vi "Automatic Teller Machine (ATM).vi"() -> ()   [LabVIEW 2025]
doc: "ATM main VI."
uses:
  Active User Data.ctl
  Queue Cluster.ctl
  States.ctl
  Account Balance Data Cluster.ctl
panel:
  in  "Enter":bool
  in  "User Input":string
  in  "Right Buttons":T1
  out "Right Menu":T2
  in  "Left Buttons":T1
  out "Left Menu":T2
  in  "Card Simulator":bool
  out "ATM Messages":string
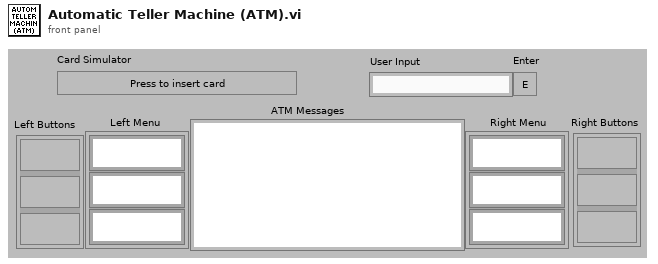
[diagram p1: front panel]
types:
  T1 = cluster{"Func Button":bool, "Func Button 2":bool, "Func Button 3":bool}
  T2 = cluster{"RFS String":string, "RFS String 2":string, "RFS String 3":string}
  T3 = typedef "Active User Data.ctl" = cluster{"Name":string, "Account Balance":dbl, "PIN":string}
  T4 = cluster{"RFS String":refnum<vi>, "RFS String 2":refnum<vi>, "RFS String 3":refnum<vi>}
  T5 = cluster{"Func Button":refnum<vi>, "Func Button 2":refnum<vi>, "Func Button 3":refnum<vi>}
  T6 = typedef "Queue Cluster.ctl" = cluster{"States":T7, "Data":variant}
  T7 = typedef "States.ctl" = enum16{"Withdraw", "Update Account Balance", "Deposit", "Balance Inquiry", "Verify Account", "Enable Account Actions", "Collect User Input", "Exit", "Init"}
  T8 = cluster{"Left Menu Strings":cluster{"RFS String":refnum<vi>, "RFS String 2":refnum<vi>, "RFS String 3":refnum<vi>}, "Right Menu Strings":cluster{"RFS String":refnum<vi>, "RFS String 2":refnum<vi>, "RFS String 3":refnum<vi>}, "Card Simulator":refnum<vi>, "Enter":refnum<vi>, "User Input":refnum<vi>, "Left Menu Button Refs":cluster{"Func Button":refnum<vi>, "Func Button 2":refnum<vi>, "Func Button 3":refnum<vi>}, "Right Menu Button Refs":cluster{"Func Button":refnum<vi>, "Func Button 2":refnum<vi>, "Func Button 3":refnum<vi>}}
  T9 = enum8{"Enabled", "Disabled", "Disabled and Grayed Out"}
  T10 = cluster{"User Input":string, "f":enum16{"Add", "Subtract"}}
  T11 = typedef "Account Balance Data Cluster.ctl" = cluster{"User Input":string, "Process":enum16{"Add", "Subtract"}}
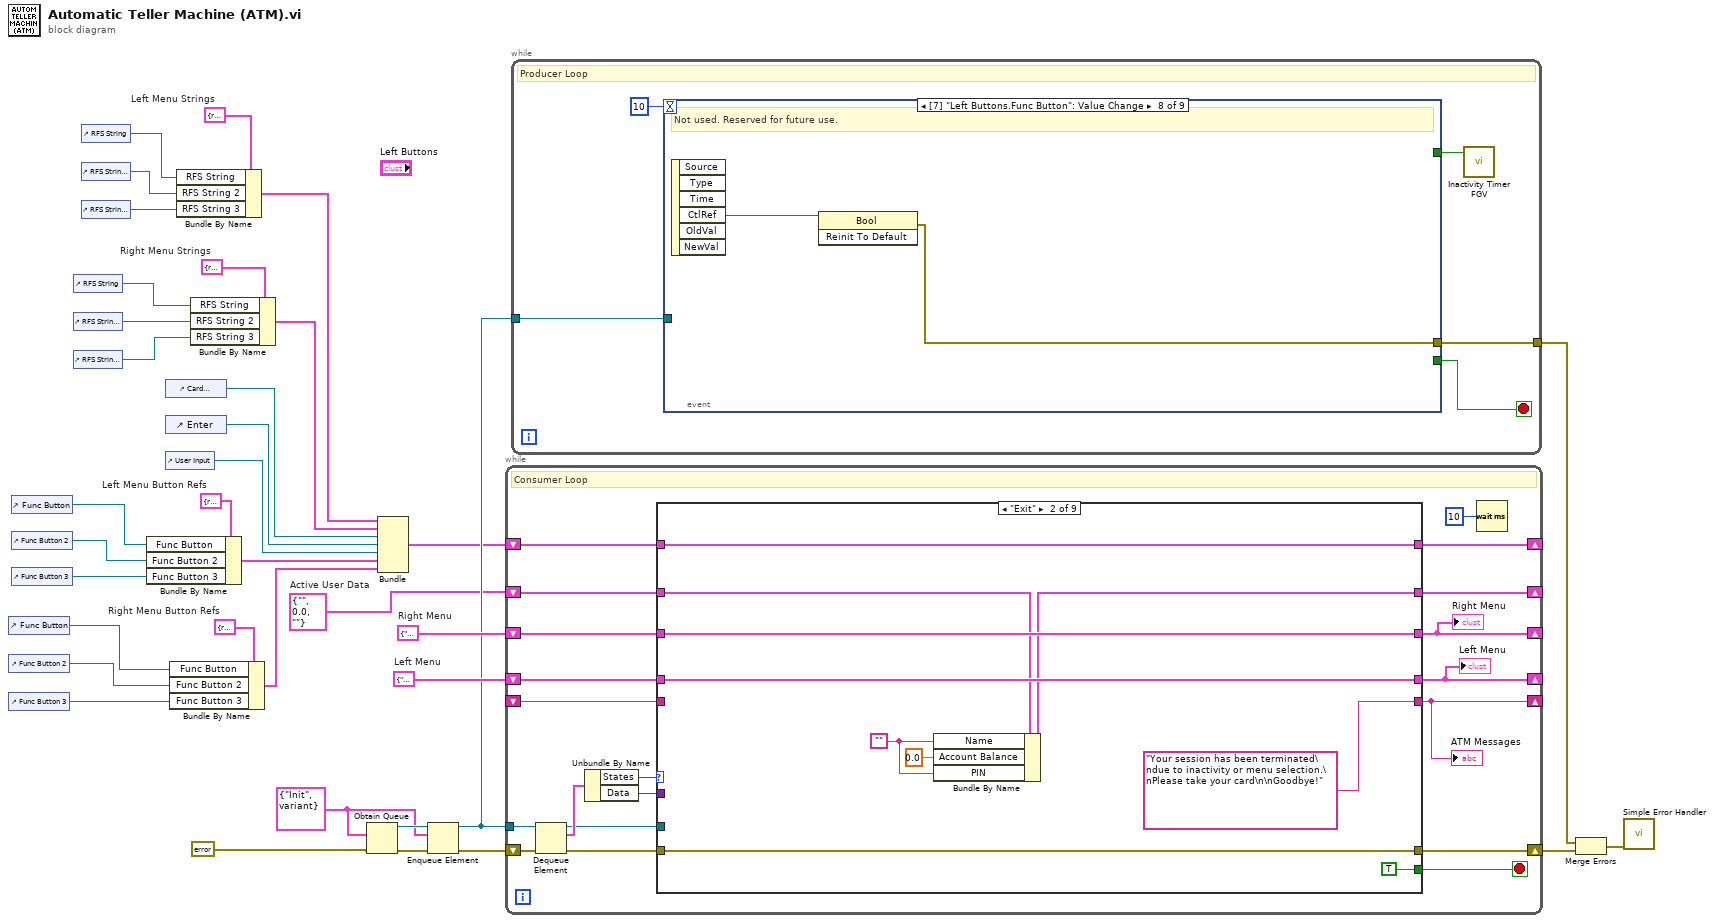
[diagram p0: block diagram]
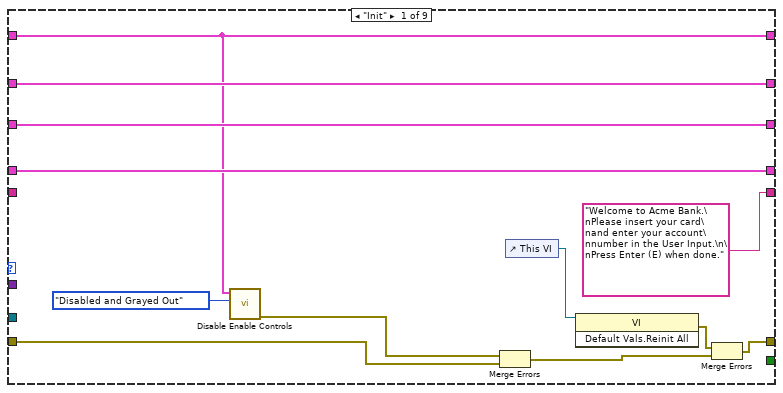
[diagram p2: hidden frame]
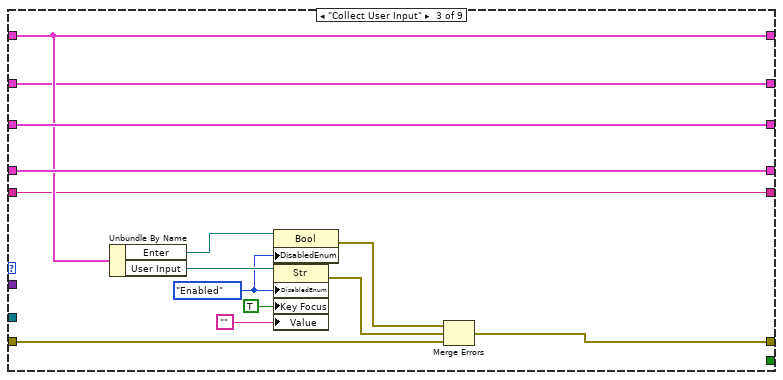
[diagram p3: hidden frame]
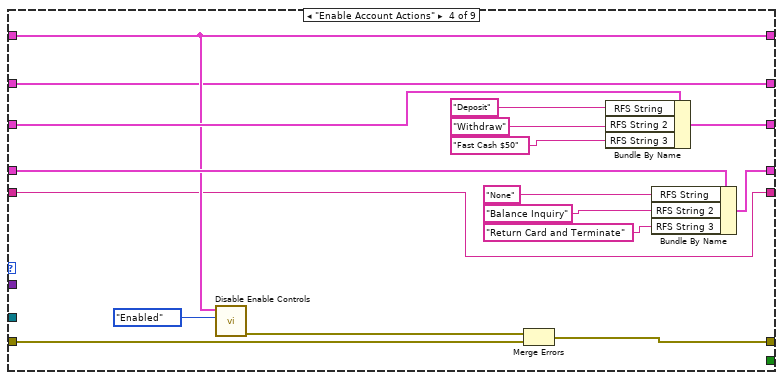
[diagram p4: hidden frame]
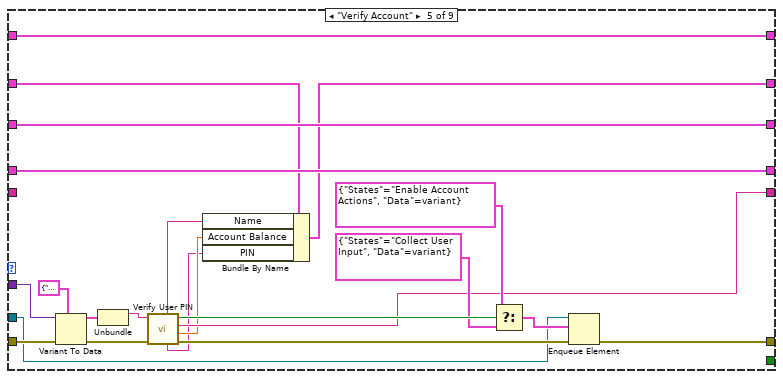
[diagram p5: hidden frame]
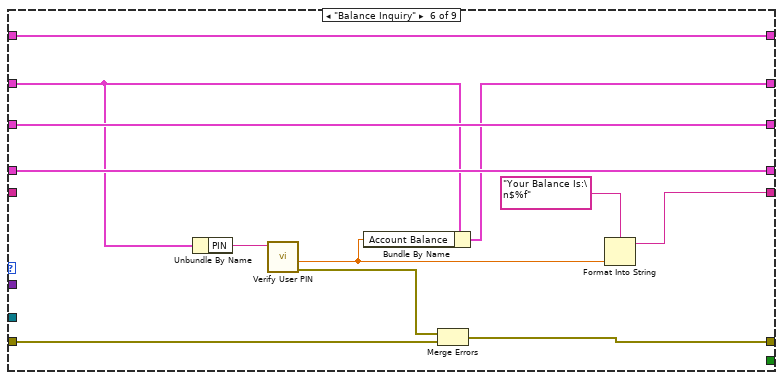
[diagram p6: hidden frame]
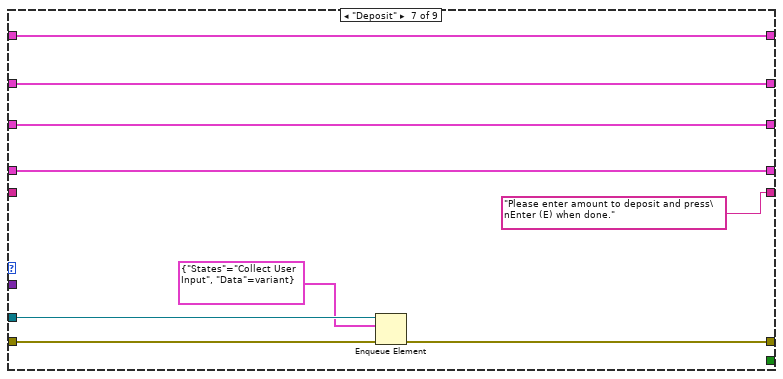
[diagram p7: hidden frame]
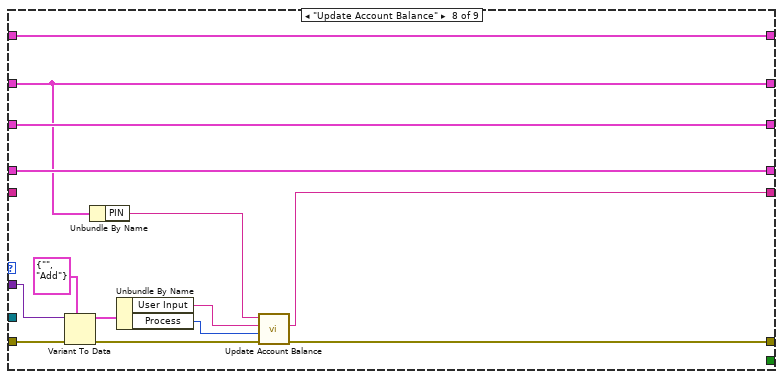
[diagram p8: hidden frame]
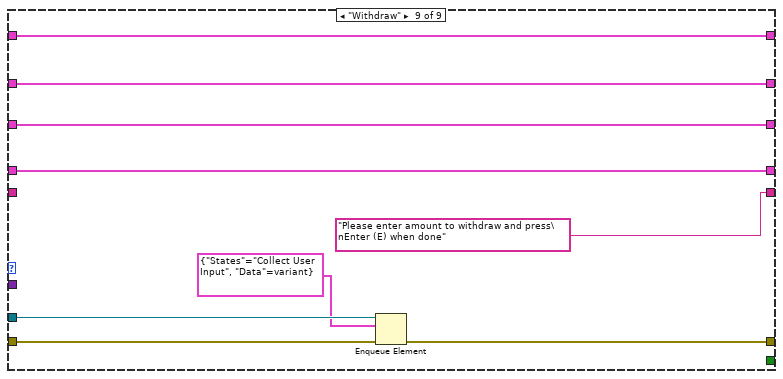
[diagram p9: hidden frame]
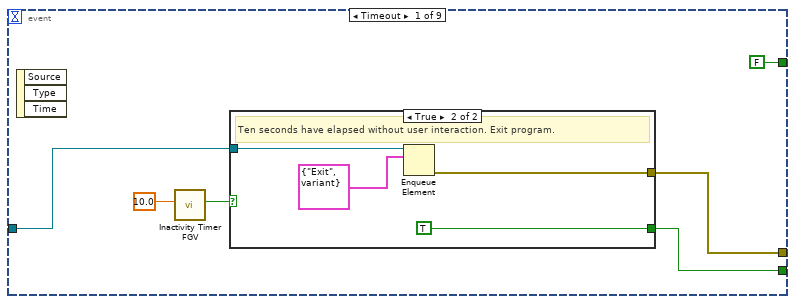
[diagram p10: hidden frame]
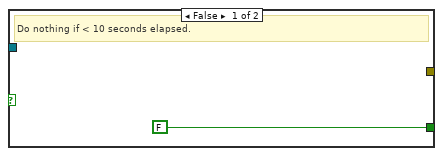
[diagram p11: hidden frame]
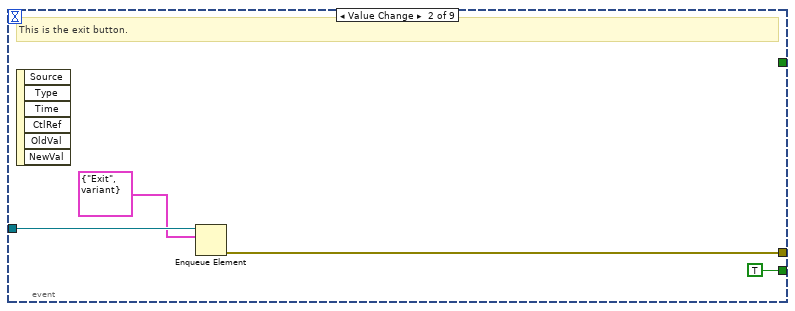
[diagram p12: hidden frame]
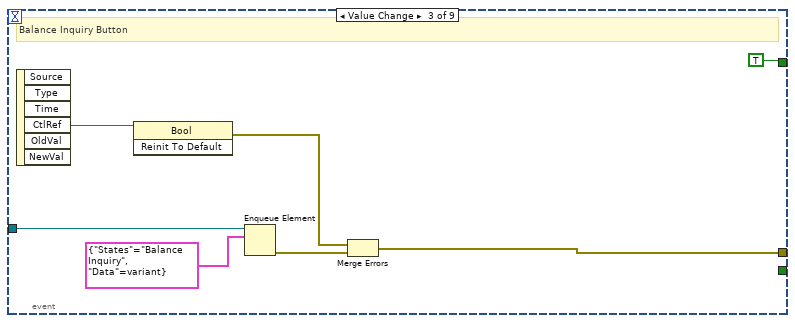
[diagram p13: hidden frame]
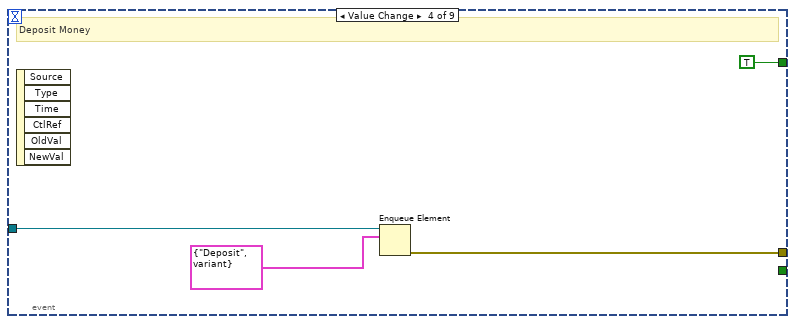
[diagram p14: hidden frame]
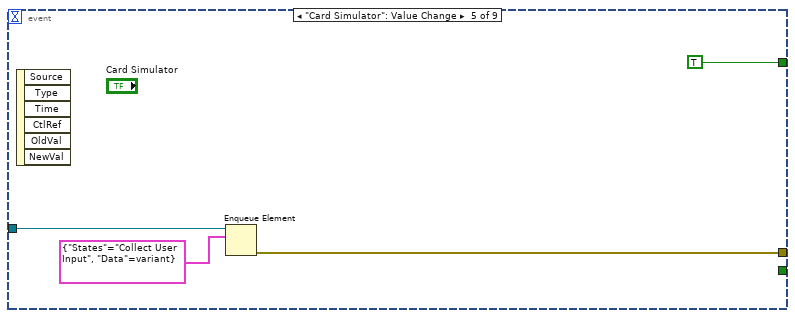
[diagram p15: hidden frame]
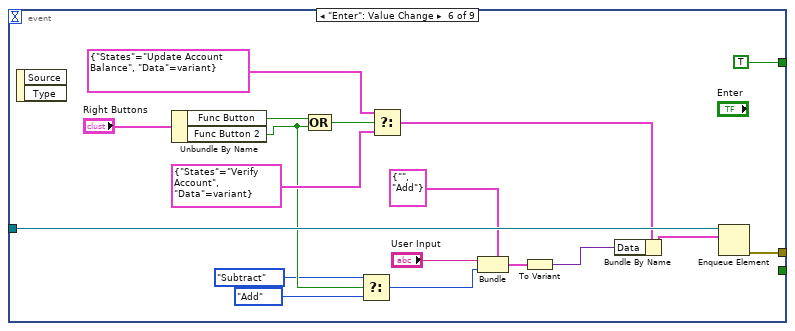
[diagram p16: hidden frame]
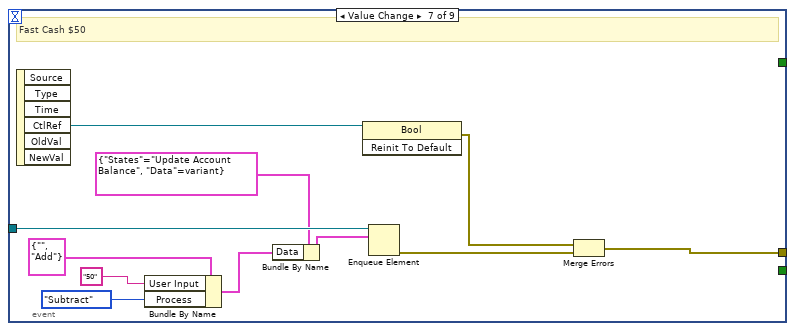
[diagram p17: hidden frame]
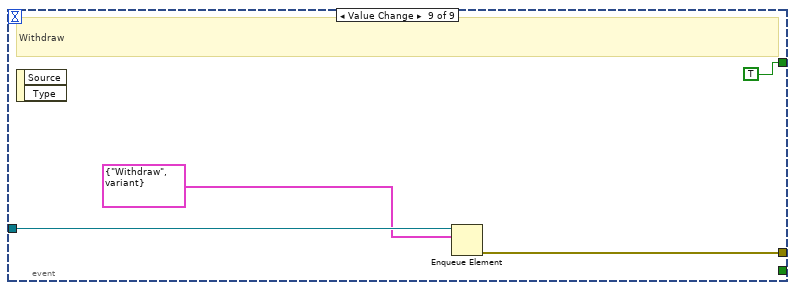
[diagram p18: hidden frame]
diagram:
  w2 = T3 {"Name"="", "Account Balance"=0.0, "PIN"=""}  # Active User Data
  w6 = T2 {"RFS String"="", "RFS String 2"="", "RFS String 3"=""}  # Left Menu
  w8 = T4 {"RFS String"=refnum, "RFS String 2"=refnum, "RFS String 3"=refnum}  # Right Menu Strings
  w13 = T4 {"RFS String"=refnum, "RFS String 2"=refnum, "RFS String 3"=refnum}  # Left Menu Strings
  w17 = T2 {"RFS String"="", "RFS String 2"="", "RFS String 3"=""}  # Right Menu
  w24 = T5 {"Func Button"=refnum, "Func Button 2"=refnum, "Func Button 3"=refnum}  # Right Menu Button Refs
  w28 = T5 {"Func Button"=refnum, "Func Button 2"=refnum, "Func Button 3"=refnum}  # Left Menu Button Refs
  w33 = T6 {"States"=enum."Init", "Data"=variant}
  n1 = control-ref of="Func Button"() -> (w27:refnum<vi>)
  n2 = control-ref of="Func Button 2"() -> (w26:refnum<vi>)
  n3 = control-ref of="Func Button 3"() -> (w25:refnum<vi>)
  n4 = control-ref of="Func Button"() -> (w30:refnum<vi>)
  n5 = control-ref of="Func Button 2"() -> (w31:refnum<vi>)
  n6 = control-ref of="Func Button 3"() -> (w29:refnum<vi>)
  n7 = control-ref of="RFS String"() -> (w11:refnum<vi>)
  n8 = control-ref of="RFS String 2"() -> (w10:refnum<vi>)
  n9 = control-ref of="RFS String 3"() -> (w9:refnum<vi>)
  n10 = control-ref of="RFS String"() -> (w16:refnum<vi>)
  n11 = control-ref of="RFS String 2"() -> (w15:refnum<vi>)
  n12 = control-ref of="RFS String 3"() -> (w14:refnum<vi>)
  n13 = Bundle By Name(cluster=w28, "Func Button"=w30, "Func Button 2"=w31, "Func Button 3"=w29) -> (w20:T5)
  n14 = control-ref of="Card Simulator"() -> (w23:refnum<vi>)
  n15 = control-ref of="Enter"() -> (w22:refnum<vi>)
  n16 = control-ref of="User Input"() -> (w21:refnum<vi>)
  n17 = Bundle By Name(cluster=w24, "Func Button"=w27, "Func Button 2"=w26, "Func Button 3"=w25) -> (w19:T5)
  n18 = Bundle By Name(cluster=w13, "RFS String"=w16, "RFS String 2"=w15, "RFS String 3"=w14) -> (w12:T4)
  n19 = Bundle By Name(cluster=w8, "RFS String"=w11, "RFS String 2"=w10, "RFS String 3"=w9) -> (w7:T4)
  n20 = Obtain Queue(element data type=w33, error in (no error)=errorcluster {"status"=FALSE, "code"=0, "source"=""}) -> (queue out=w36:refnum<queue>, error out=w35:errorcluster)  [unwired: 3 in, 1 out]
  n21 = Bundle("Left Menu Strings"=w12, "Right Menu Strings"=w7, "Card Simulator"=w23, "Enter"=w22, "User Input"=w21, "Left Menu Button Refs"=w20, "Right Menu Button Refs"=w19) -> (w1:T8)  [unwired: 1 in]
  n22 = Enqueue Element(queue=w36, element=w33, error in (no error)=w35) -> (queue out=w5:refnum<queue>, error out=w4:errorcluster)  [unwired: 1 in, 1 out]
  n23 = while {
    tunnel: w5 -> [w53]
    shift-right: [w48] -> _
    shift-left: w1 -> [w39]
    shift-right: [w46] -> _
    shift-left: w6 -> [w47]
    shift-right: [w44] -> _
    shift-left: w17 -> [w45]
    shift-right: [w42] -> _
    shift-left: _ -> [w41]
    shift-right: [w55] -> w34
    shift-left: w4 -> [w56]
    shift-right: [w37] -> _
    shift-left: w2 -> [w38]
    stop <- w49 stop-if-true
    # "Consumer Loop"
    n24 = Dequeue Element(queue=w53, error in (no error)=w56) -> (queue out=w43:refnum<queue>, element=w52:T6, error out=w54:errorcluster)  [unwired: 1 in, 1 out]
    n25 = Unbundle By Name(w52) -> ("States"=w51:T7, "Data"=w50:variant)
    n26 = case shown="\"Exit\"" w51 {
      tunnel: w54 -> [w68 w73 w92 w109 w128 w143 w152 w166 w175]
      tunnel: [w66 w73 w81 w97 w119 w135 w146 w158 w169] -> w55
      tunnel: w50 -> [_ _ _ _ w126 _ _ w162 _]
      tunnel: [_ TRUE _ _ _ _ _ _ _] -> w49
      tunnel: ["Welcome to Acme Bank.\nPlease insert your card\nand enter your account\nnumber in the User Input.\n\nPress Enter (E) when done." "Your session has been terminated\ndue to inactivity or menu selection.\nPlease take your card\n\nGoodbye!" w83 w95 w118 w139 "Please enter amount to deposit and press\nEnter (E) when done." ("ATM Message") w154 "Please enter amount to withdraw and press\nEnter (E) when done" ("ATM Message")] -> w42
      tunnel: w39 -> [w59 w76 w89 w98 w131 w138 w147 w165 w174]
      tunnel: [w59 w76 w89 w98 w131 w138 w147 w165 w174] -> w48
      tunnel: w47 -> [w65 w75 w91 w108 w130 w142 w151 w164 w173]
      tunnel: [w65 w75 w91 w104 w130 w142 w151 w164 w173] -> w46
      tunnel: w45 -> [w64 w74 w90 w103 w129 w141 w150 w163 w172]
      tunnel: [w64 w74 w90 w99 w129 w141 w150 w163 w172] -> w44
      tunnel: w43 -> [_ _ _ _ w120 _ w145 _ w168]
      tunnel: w41 -> [_ _ w83 w95 _ _ _ _ _]
      tunnel: w38 -> [w60 w72 w82 w94 w117 w137 w149 w161 w171]
      tunnel: [w60 w71 w82 w94 w116 w133 w149 w161 w171] -> w37
      frame "Init" {
        n27 = call "Disable Enable Controls.vi"("Disable or Enable"=T9."Disabled and Grayed Out", "Cluster"=w59) -> ("error out"=w57:errorcluster)  [unwired: 9 in]
        n28 = Merge Errors(w57, w68) -> (w61:errorcluster)
        n29 = control-ref of="This VI"() -> (w63:refnum<vi>)
        n30 = invoke on="Invoke Node" class="VI" method="Default Vals.Reinit All"(reference=w63) -> (error out=w62:errorcluster)  [unwired: 2 in, 2 out]
        n31 = Merge Errors(w62, w61) -> (w66:errorcluster)
      }
      frame "Exit" {
        w70 = "" ("Name")
        n32 = Bundle By Name(cluster=w72, "Name"=w70, "Account Balance"=0.0, "PIN"=w70) -> (w71:T3)
      }
      frame "Collect User Input" {
        w85 = T9."Enabled" ("Disabled")
        n33 = Unbundle By Name(w89) -> ("Enter"=w86:refnum<vi>, "User Input"=w88:refnum<vi>)
        n34 = property on="Property Node" class="Bool"(reference=w86, "DisabledEnum"=w85) -> (error out=w79:errorcluster)  [unwired: 1 in, 1 out]
        n35 = property on="Property Node" class="Str"(reference=w88, "DisabledEnum"=w85, "Key Focus"=TRUE ("Selected"), "Value"="" ("Empty String Constant")) -> (error out=w80:errorcluster)  [unwired: 1 in, 1 out]
        n36 = Merge Errors(w79, w80, w92) -> (w81:errorcluster)
      }
      frame "Enable Account Actions" {
        n37 = call "Disable Enable Controls.vi"("Disable or Enable"=T9."Enabled", "Cluster"=w98) -> ("error out"=w96:errorcluster)  [unwired: 9 in]
        n38 = Merge Errors(w96, w109) -> (w97:errorcluster)
        n39 = Bundle By Name(cluster=w103, "RFS String"="Deposit" ("Right Menu.RFS String"), "RFS String 2"="Withdraw" ("Right Menu.RFS String 2"), "RFS String 3"="Fast Cash $50" ("Right Menu.RFS String 3")) -> (w99:T2)
        n40 = Bundle By Name(cluster=w108, "RFS String"="None" ("Left Menu.RFS String"), "RFS String 2"="Balance Inquiry" ("Left Menu.RFS String 2"), "RFS String 3"="Return Card and Terminate" ("Left Menu.RFS String 3")) -> (w104:T2)
      }
      frame "Verify Account" {
        n41 = Variant To Data(error in=w128, type=T10 {"User Input"="", "f"=enum."Add"} ("cluster"), Variant=w126) -> (data=w111:T10, error out=w127:errorcluster)
        n42 = Unbundle(w111) -> ("User Input"=w110:string)  [unwired: 1 out]
        n43 = call "Verify User PIN.vi"("error in (no error)"=w127, "PIN"=w110) -> ("error out"=w121:errorcluster, "Account Balance"=w114:dbl, "ATM Message"=w118:string, "Verified?"=w124:bool, "User PIN"=w113:string, "Account Holder"=w115:string)  [unwired: 4 in]
        n44 = Bundle By Name(cluster=w117, "Name"=w115, "Account Balance"=w114, "PIN"=w113) -> (w116:T3)
        n45 = Select(t=T6 {"States"=enum."Enable Account Actions", "Data"=variant}, s=w124, f=T6 {"States"=enum."Collect User Input", "Data"=variant}) -> (s? t:f=w122:T6)
        n46 = Enqueue Element(queue=w120, element=w122, error in (no error)=w121) -> (error out=w119:errorcluster)  [unwired: 1 in, 2 out]
      }
      frame "Balance Inquiry" {
        n47 = Unbundle By Name(w137) -> ("PIN"=w136:string)
        n48 = call "Verify User PIN.vi"("PIN"=w136) -> ("error out"=w134:errorcluster, "Account Balance"=w132:dbl)  [unwired: 5 in, 4 out]
        n49 = Bundle By Name(cluster=w137, "Account Balance"=w132) -> (w133:T3)
        n50 = Merge Errors(w134, w143) -> (w135:errorcluster)
        n51 = Format Into String(format string="Your Balance Is:\n$%f", w132) -> (resulting string=w139:string)  [unwired: 2 in, 1 out]
      }
      frame "Deposit" {
        n52 = Enqueue Element(queue=w145, element=T6 {"States"=enum."Collect User Input", "Data"=variant}, error in (no error)=w152) -> (error out=w146:errorcluster)  [unwired: 1 in, 2 out]
      }
      frame "Update Account Balance" {
        n53 = Variant To Data(error in=w166, type=T11 {"User Input"="", "Process"=enum."Add"} ("Update Account Balance Data Cluster"), Variant=w162) -> (data=w157:T11, error out=w159:errorcluster)
        n54 = Unbundle By Name(w161) -> ("PIN"=w160:string)
        n55 = Unbundle By Name(w157) -> ("User Input"=w155:string, "Process"=w156:enum16{"Add", "Subtract"})
        n56 = call "Update Account Balance.vi"("error in (no error)"=w159, "Add or Subtract"=w156, "Amount"=w155, "PIN"=w160) -> ("error out"=w158:errorcluster, "Message"=w154:string)  [unwired: 6 in]
      }
      frame "Withdraw" {
        n57 = Enqueue Element(queue=w168, element=T6 {"States"=enum."Collect User Input", "Data"=variant}, error in (no error)=w175) -> (error out=w169:errorcluster)  [unwired: 1 in, 2 out]
      }
    }
    "ATM Messages" <- w42
    "Left Menu" <- w46
    "Right Menu" <- w44
    n58 = Wait (ms)(milliseconds to wait=u32 10) -> ()  [unwired: 1 out]
  }
  n59 = while {
    tunnel: w5 -> [w179]
    tunnel: [w180] -> w32
    stop <- w177 stop-if-true
    # "Producer Loop"
    n60 = event shown="[7] \"Left Buttons.Func Button\": Value Change" {
      selector: _ -> [_ _ _ _ _ _ _ _ _]
      dyn-events: _ -> [_ _ _ _ _ _ _ _ _]
      timeout: 10 -> [_ _ _ _ _ _ _ _ _]
      tunnel: w179 -> [w184 w195 w202 w206 w210 w228 w239 _ w245]
      tunnel: [w183 w193 w197 w205 w209 w227 w230 w240 w244] -> w180
      tunnel: [w182 TRUE _ _ _ _ _ _ _] -> w177
      tunnel: [FALSE ("Reset") _ TRUE ("Reset") TRUE ("Reset") TRUE ("Reset") TRUE ("Reset") _ _ TRUE ("Reset")] -> w176
      event Timeout {
        n61 = event-data() -> ()  [unwired: 1 in, 3 out]
        n62 = call "Inactivity Timer FGV.vi"("Time Target (s)"=10.0) -> ("Time has Elapsed"=w186:bool)  [unwired: 9 in, 1 out]
        n63 = case shown="True" w186 {
          tunnel: [FALSE TRUE] -> w182
          tunnel: w184 -> [_ w191]
          tunnel: [_ w189] -> w183
          frame False {
            # "Do nothing if < 10 seconds elapsed."
          }
          frame True {
            # "Ten seconds have elapsed without user interaction. Exit program."
            n64 = Enqueue Element(queue=w191, element=T6 {"States"=enum."Exit", "Data"=variant}) -> (error out=w189:errorcluster)  [unwired: 2 in, 2 out]
          }
        }
      }
      event "Left Buttons.Func Button 3": Value Change {
        # "This is the exit button."
        n65 = event-data() -> ()  [unwired: 1 in, 6 out]
        n66 = Enqueue Element(queue=w195, element=T6 {"States"=enum."Exit", "Data"=variant} ("Queue Cluster")) -> (error out=w193:errorcluster)  [unwired: 2 in, 2 out]
      }
      event "Left Buttons.Func Button 2": Value Change {
        # "Balance Inquiry Button"
        n67 = event-data() -> ("CtlRef"=w198:refnum<vi>)  [unwired: 1 in, 5 out]
        n68 = invoke on="Invoke Node" class="Bool" method="Reinit To Default"(reference=w198) -> (error out=w196:errorcluster)  [unwired: 2 in, 2 out]
        n69 = Enqueue Element(queue=w202, element=T6 {"States"=enum."Balance Inquiry", "Data"=variant}) -> (error out=w201:errorcluster)  [unwired: 2 in, 2 out]
        n70 = Merge Errors(w196, w201) -> (w197:errorcluster)
      }
      event "Right Buttons.Func Button": Value Change {
        # "Deposit Money"
        n71 = event-data() -> ()  [unwired: 1 in, 6 out]
        n72 = Enqueue Element(queue=w206, element=T6 {"States"=enum."Deposit", "Data"=variant}) -> (error out=w205:errorcluster)  [unwired: 2 in, 2 out]
      }
      event "Card Simulator": Value Change {
        n73 = event-data() -> ()  [unwired: 1 in, 6 out]
        n74 = Enqueue Element(queue=w210, element=T6 {"States"=enum."Collect User Input", "Data"=variant}) -> (error out=w209:errorcluster)  [unwired: 2 in, 2 out]
      }
      event "Enter": Value Change {
        n75 = event-data() -> ()  [unwired: 1 in, 2 out]
        n76 = Unbundle By Name("Right Buttons") -> ("Func Button"=w222:bool, "Func Button 2"=w216:bool)
        n77 = Compound Arithmetic op=OR(w222, w216) -> (w221:bool)
        n78 = Select(t=enum16{"Add", "Subtract"}."Subtract" ("Add or Subtract"), s=w216, f=enum16{"Add", "Subtract"}."Add") -> (s? t:f=w213:enum16{"Add", "Subtract"})
        n79 = Select(t=T6 {"States"=enum."Update Account Balance", "Data"=variant}, s=w221, f=T6 {"States"=enum."Verify Account", "Data"=variant}) -> (s? t:f=w218:T6)
        n80 = Bundle(cluster=T11 {"User Input"="", "Process"=enum."Add"} ("Update Account Balance Data Cluster"), "User Input"="User Input", "Process"=w213) -> (w217:T11)
        n81 = To Variant(anything=w217) -> (Variant=w225:variant)
        n82 = Bundle By Name(cluster=w218, "Data"=w225) -> (w226:T6)
        n83 = Enqueue Element(queue=w228, element=w226) -> (error out=w227:errorcluster)  [unwired: 2 in, 2 out]
      }
      event "Right Buttons.Func Button 3": Value Change {
        # "Fast Cash $50"
        n84 = event-data() -> ("CtlRef"=w231:refnum<vi>)  [unwired: 1 in, 5 out]
        n85 = Bundle By Name(cluster=T11 {"User Input"="", "Process"=enum."Add"}, "User Input"="50", "Process"=enum16{"Add", "Subtract"}."Subtract" ("f")) -> (w232:T11)
        n86 = Bundle By Name(cluster=T6 {"States"=enum."Update Account Balance", "Data"=variant}, "Data"=w232) -> (w233:T6)
        n87 = invoke on="Invoke Node" class="Bool" method="Reinit To Default"(reference=w231) -> (error out=w229:errorcluster)  [unwired: 2 in, 2 out]
        n88 = Enqueue Element(queue=w239, element=w233) -> (error out=w238:errorcluster)  [unwired: 2 in, 2 out]
        n89 = Merge Errors(w229, w238) -> (w230:errorcluster)
      }
      event "Left Buttons.Func Button": Value Change {
        # "Not used. Reserved for future use."
        n90 = event-data() -> ("CtlRef"=w241:refnum<vi>)  [unwired: 1 in, 5 out]
        n91 = invoke on="Invoke Node" class="Bool" method="Reinit To Default"(reference=w241) -> (error out=w240:errorcluster)  [unwired: 2 in, 2 out]
      }
      event "Right Buttons.Func Button 2": Value Change {
        # "Withdraw"
        n92 = event-data() -> ()  [unwired: 1 in, 2 out]
        n93 = Enqueue Element(queue=w245, element=T6 {"States"=enum."Withdraw", "Data"=variant}) -> (error out=w244:errorcluster)  [unwired: 2 in, 2 out]
      }
    }
    n94 = call "Inactivity Timer FGV.vi"("Reset"=w176) -> ()  [unwired: 9 in, 2 out]
  }
  n95 = Merge Errors(w32, w34) -> (w3:errorcluster)
  n96 = call <vilib>:"Simple Error Handler.vi"("error in (no error)"=w3) -> ()  [unwired: 4 in, 5 out]
